vi "Get Key.vi"(1 "Key Code":i16) -> (0 "Key":string)   [LabVIEW 2021, in "Seq Edit Quick Drop.lvlib"]
uses:
  Seq Edit Quick Drop.lvlib
  Key Codes Constants.vi
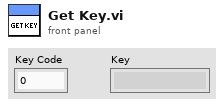
[diagram p1: front panel]
types:
  T1 = typedef "Seq Edit Quick Drop.lvlib/Key Codes Constants.ctl" = cluster{"Code":i16, "Key":string}[]
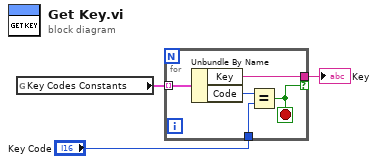
[diagram p0: block diagram]
diagram:
  n1 = global read "Key Codes Constants.vi" "Key Codes Constants"() -> (w1:T1)
  n2 = for {
    tunnel: w1 -> [w8] mode=indexing
    tunnel: [w7] -> w2 if=w6
    tunnel: "Key Code" -> [w5]
    stop <- w6 stop-if-true
    n3 = Unbundle By Name(w8) -> ("Key"=w7:string, "Code"=w4:i16)
    n4 = Equal?(x=w4, y=w5) -> (x = y?=w6:bool)
  }
  "Key" <- w2
